vi "InjectFaults.vi"(0 "MotorMeasurements":T1, 5 "Fault Injection":T2, 7 "Safety Current Trip":dbl, 9 "Safety Temperature Trip":dbl, 11 "Safety Vibration Trip":dbl) -> (4 "Modified Measurements":T1, 15 "Injected System Fault":bool)   [LabVIEW 2026]
uses:
  MotorMeasurements.ctl
  FaultInjectionMode.ctl
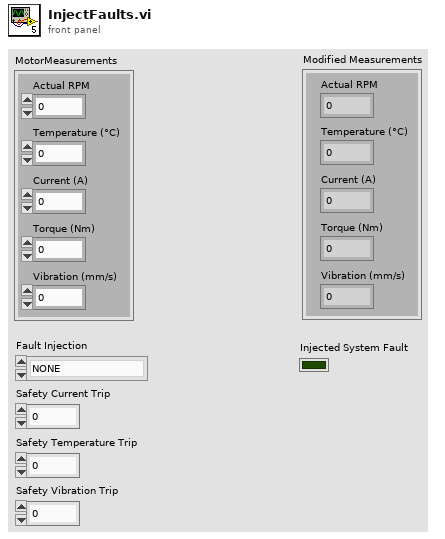
[diagram p1: front panel]
types:
  T1 = typedef "MotorMeasurements.ctl" = cluster{"Temperature (°C)":dbl, "Current (A)":dbl, "Torque (Nm)":dbl, "Vibration (mm/s)":dbl, "Actual RPM":dbl}
  T2 = typedef "FaultInjectionMode.ctl" = enum16{"NONE", "OVERCURRENT", "OVERTEMPERATURE", "HIGH_VIBRATION", "RPM_SENSOR_FAILURE"}
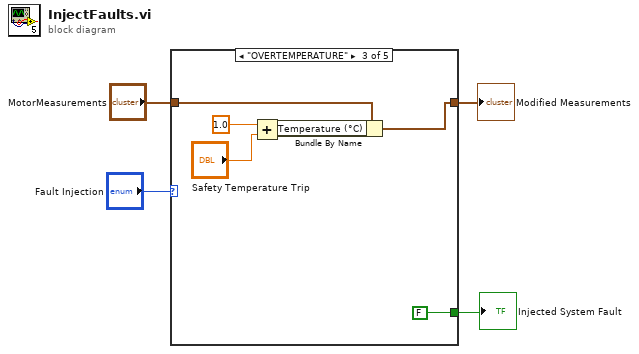
[diagram p0: block diagram]
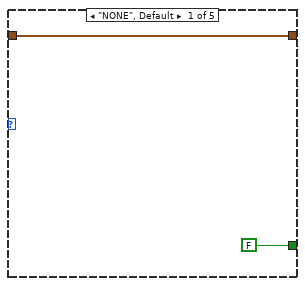
[diagram p2: hidden frame]
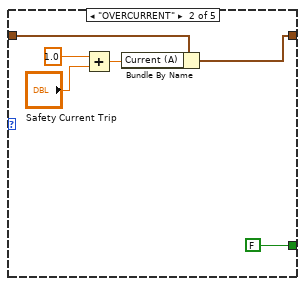
[diagram p3: hidden frame]
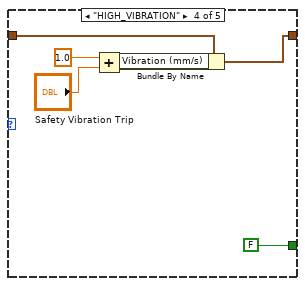
[diagram p4: hidden frame]
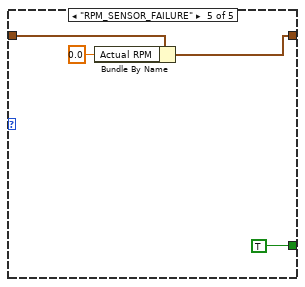
[diagram p5: hidden frame]
diagram:
  n1 = case shown="\"OVERTEMPERATURE\"" "Fault Injection" {
    tunnel: "MotorMeasurements" -> [w6 w12 w16 w21 w28]
    tunnel: [w6 w7 w14 w19 w26] -> w2
    tunnel: [FALSE FALSE FALSE FALSE TRUE] -> w1
    frame "NONE", Default {
    }
    frame "OVERCURRENT" {
      n2 = Add(x=1.0, y="Safety Current Trip") -> (x+y=w11:dbl)
      n3 = Bundle By Name(cluster=w12, "Current (A)"=w11) -> (w7:T1)
    }
    frame "OVERTEMPERATURE" {
      n4 = Add(x=1.0, y="Safety Temperature Trip") -> (x+y=w18:dbl)
      n5 = Bundle By Name(cluster=w16, "Temperature (°C)"=w18) -> (w14:T1)
    }
    frame "HIGH_VIBRATION" {
      n6 = Add(x=1.0, y="Safety Vibration Trip") -> (x+y=w23:dbl)
      n7 = Bundle By Name(cluster=w21, "Vibration (mm/s)"=w23) -> (w19:T1)
    }
    frame "RPM_SENSOR_FAILURE" {
      n8 = Bundle By Name(cluster=w28, "Actual RPM"=0.0) -> (w26:T1)
    }
  }
  "Modified Measurements" <- w2
  "Injected System Fault" <- w1
